vi "Clase labview.vi"() -> ()   [LabVIEW 2019]
panel:
  out "arctan(x)":dbl
  out "arccos(x)":dbl
  in  "ADYACENTE":dbl
  out "arcsin(x)":dbl
  in  "HIPOTENUSA":dbl
  in  "OPUESTO":dbl
  out "Numeric":dbl
  in  "Boolean 3":bool
  in  "Boolean 2":bool
  in  "Boolean":bool
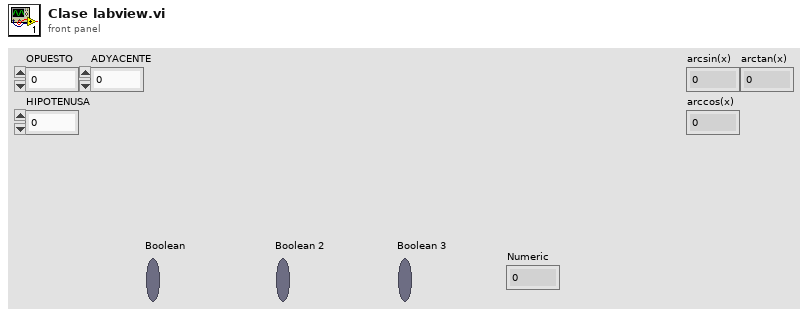
[diagram p1: front panel]
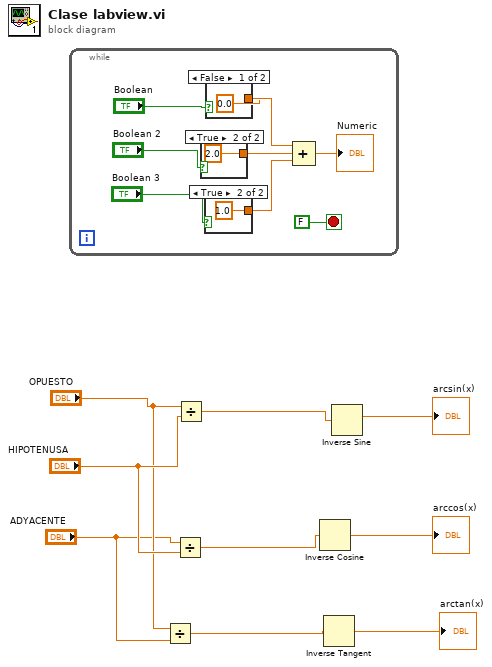
[diagram p0: block diagram]
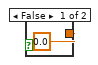
[diagram p2: hidden frame]
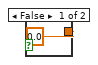
[diagram p3: hidden frame]
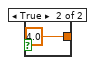
[diagram p4: hidden frame]
diagram:
  n1 = while {
    stop <- FALSE stop-if-true
    n2 = case shown="True" "Boolean 2" {
      tunnel: [0.0 2.0] -> w16
      frame False {
      }
      frame True {
      }
    }
    n3 = case shown="True" "Boolean 3" {
      tunnel: [0.0 1.0] -> w15
      frame False {
      }
      frame True {
      }
    }
    n4 = case shown="False" "Boolean" {
      tunnel: [0.0 4.0] -> w17
      frame False {
      }
      frame True {
      }
    }
    n5 = Compound Arithmetic op=ADD(w17, w16, w15) -> (→"Numeric":dbl)
  }
  n6 = Divide(x="OPUESTO", y="ADYACENTE") -> (x/y=w3:dbl)
  n7 = Divide(x="ADYACENTE", y="HIPOTENUSA") -> (x/y=w4:dbl)
  n8 = Divide(x="OPUESTO", y="HIPOTENUSA") -> (x/y=w9:dbl)
  n9 = Inverse Cosine(1:w4) -> (0:→"arccos(x)":dbl)
  n10 = Inverse Tangent(1:w3) -> (0:→"arctan(x)":dbl)
  n11 = Inverse Sine(1:w9) -> (0:→"arcsin(x)":dbl)
